vi "读取位置.vi"(8 "error in (no error)":errorcluster caption="错误输入（无错误）", 11 "RandomMoveBool输入":refnum<class "RandomMoveBool.lvclass">) -> (0 "error out":errorcluster caption="错误输出", 2 "Position":T1 caption="位置", 3 "RandomMoveBool输出":refnum<class "RandomMoveBool.lvclass">)   [LabVIEW 2018, in "RandomMoveBool.lvclass"]
uses:
  RandomMoveBool.lvclass
  <vilib>/Utility/miscctls.llb/LVPositionTypeDef.ctl
  RandomMoveBool.lvclass/RandomMoveBool.ctl
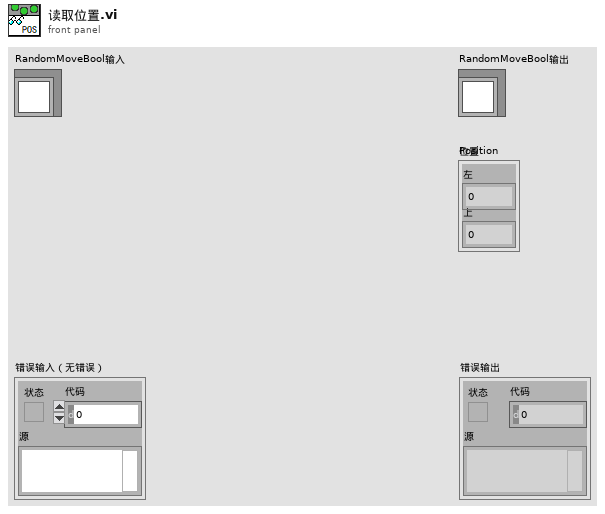
[diagram p1: front panel]
types:
  T1 = typedef "LVPositionTypeDef.ctl" = cluster{"Left":i32, "Top":i32}
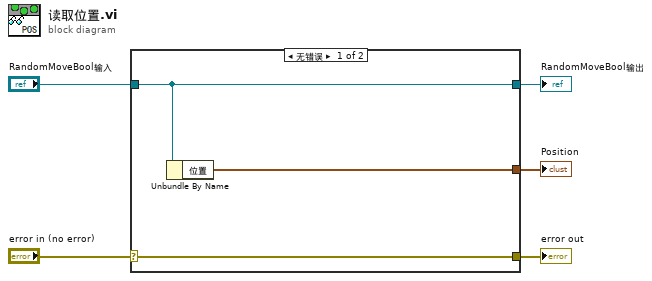
[diagram p0: block diagram]
diagram:
  n1 = case shown="无错误" "error in (no error)" {
    selector: "error in (no error)" -> [w8 w9]
    tunnel: [w8 w9] -> w4
    tunnel: [w7 w10] -> w2
    tunnel: "RandomMoveBool输入" -> [w7 w10]
    tunnel: [w6 _] -> w1
    frame No Error {
      n2 = Unbundle By Name(w7) -> ("位置"=w6:T1)
    }
    frame Error {
    }
  }
  "error out" <- w4
  "RandomMoveBool输出" <- w2
  "Position" <- w1
